vi "Feet to Encoder.vi"(11 "Distance (ft)":dbl format="%#_13g") -> (3 "Encoder Units":dbl format="%#_13g")   [LabVIEW 2016]
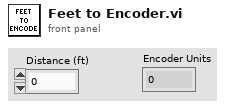
[diagram p1: front panel]
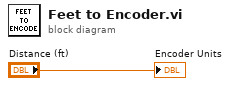
[diagram p0: block diagram]
diagram:
  "Encoder Units" <- "Distance (ft)"
